vi "Chirp signal spectrum analysis.vi"() -> ()   [LabVIEW 2019]
uses:
  <vilib>/measure/maspectr.llb/FFT Power Spectrum and PSD for 1 Chan (CDB).vi
  <vilib>/measure/NI_MAPro.lvlib
panel:
  in  "Sideband":enum16{"Lower sideband", "Upper sideband"}(ring)
  in  "Save data":bool
  in  "fs":dbl=3072000000.0 format="%#_6p"
  out "Spectrum":cluster{"f0":dbl, "df":dbl, "magnitude":dbl[]}(graph)
  out "Waveform":waveform(dbl)(graph)
  in  "N":i32=30720 format="%.0p"
  in  "f2":dbl=1000000000.0 format="%#_6p"
  in  "f1":dbl
  out "t":dbl=1e-05 format="%#_6p"
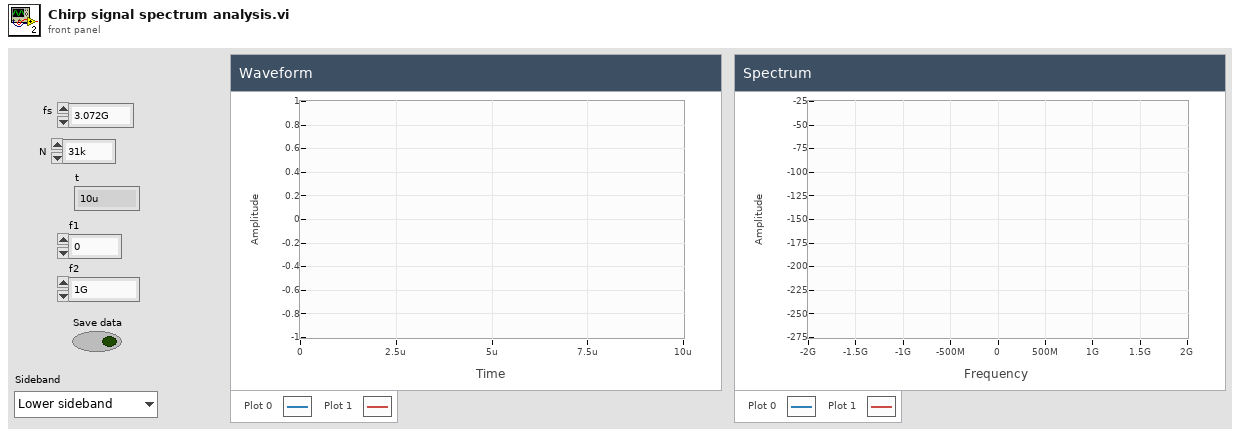
[diagram p1: front panel]
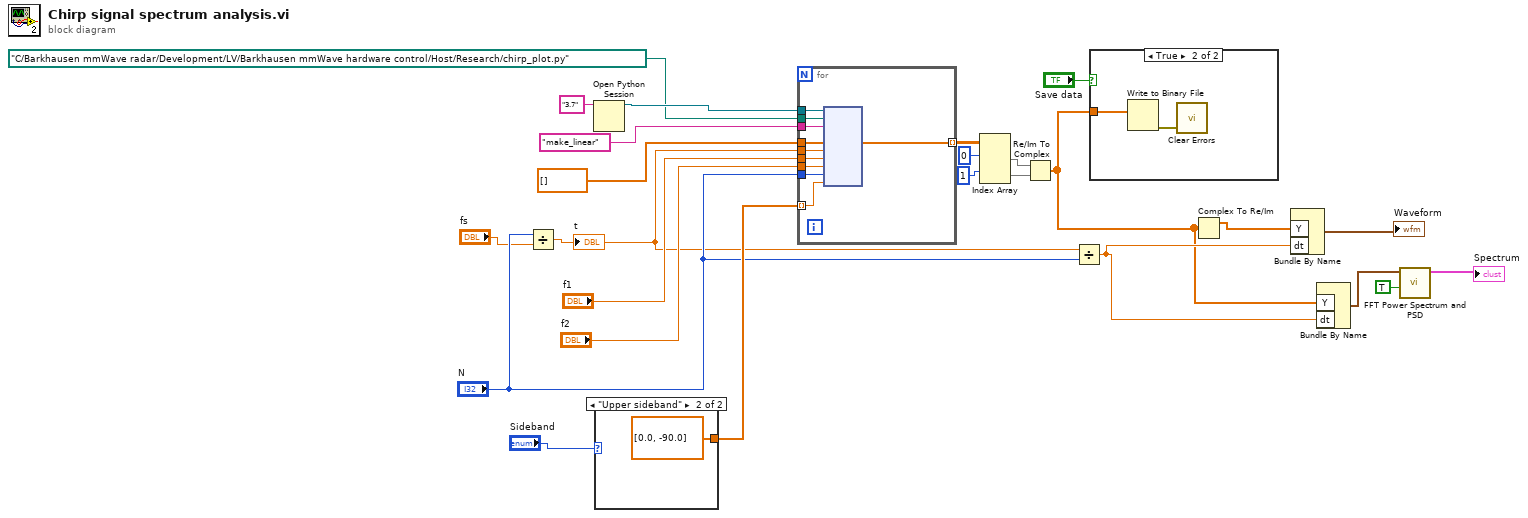
[diagram p0: block diagram]
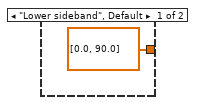
[diagram p2: hidden frame]
diagram:
  n1 = Divide(x="N", y="fs") -> (x/y=w3:dbl)
  "t" <- w3
  n2 = Open Python Session(python version="3.7" ("Python version")) -> (session out=w24:refnum<k35>)  [unwired: 2 in, 1 out]
  n3 = case shown="\"Upper sideband\"" "Sideband" {
    tunnel: [dbl[] [0.0, 90.0] ("Waveform Graph - Dark") dbl[] [0.0, -90.0] ("Waveform Graph - Dark")] -> w8
    frame "Lower sideband", Default {
    }
    frame "Upper sideband" {
    }
  }
  n4 = for {
    tunnel: w24 -> [w37]
    tunnel: path "C:/Barkhausen mmWave radar/Development/LV/Barkhausen mmWave hardware control/Host/Research/chirp_plot.py" ("module path") -> [w36]
    tunnel: "make_linear" ("function name") -> [w35]
    tunnel: "f1" -> [w34]
    tunnel: "f2" -> [w33]
    tunnel: dbl[] [] ("Waveform Graph - Dark") -> [w32]
    tunnel: w3 -> [w31]
    tunnel: "N" -> [w30]
    tunnel: [w29] -> w15 mode=indexing
    tunnel: w8 -> [w28] mode=indexing
    n5 = node(w37, w36, w35, w32, w31, w34, w33, w30, w28) -> (w29:dbl[])  [unwired: 6 in, 4 out]
  }
  n6 = Index Array(array=w15, index (row) #1=0 ("index (row)"), index (row) #2=1 ("index (row)")) -> (element #1=w11:dbl[], element #2=w12:dbl[])  [unwired: 2 in]
  n7 = Re/Im To Complex(1:w12, 2:w11) -> (0:w6:cdb[])
  n8 = Divide(x=w3, y="N") -> (x/y=w14:dbl)
  n9 = case shown="True" "Save data" {
    tunnel: w6 -> [_ w39]
    frame False {
    }
    frame True {
      n10 = Write to Binary File(data=w39) -> (error out=w38:errorcluster)  [unwired: 5 in, 2 out]
      n11 = call <vilib>:"Clear Errors.vi"("error in (no error)"=w38) -> ()  [unwired: 5 in, 2 out]
    }
  }
  n12 = Complex To Re/Im(x + iy=w6) -> (x=w7:dbl[])  [unwired: 1 out]
  n13 = Bundle By Name("Y"=w7, "dt"=w14) -> (→"Waveform":waveform(dbl))  [unwired: 1 in]
  n14 = Bundle By Name("Y"=w6, "dt"=w14) -> (w13:waveform(cdb))  [unwired: 1 in]
  n15 = call-poly <vilib>:"FFT Power Spectrum and PSD.vi"("dB On (F)"=TRUE, "time signal"=w13) -> ("Power Spectrum / PSD"=→"Spectrum":cluster{"f0":dbl, "df":dbl, "magnitude":dbl[]})  [unwired: 6 in, 3 out]
